vi "Facade.vi"(0 "Data In":T4, 2 "Display State In":T2, 3 "Container State":T3) -> (6 "Data Out":T4, 7 "Display State Out":T2, 8 "Action":T1)   [LabVIEW 2020, in "Recipe Entry.xctl"]
uses:
  Recipe Entry.xctl
  Data.ctl
  <vilib>/_xctls/Container State.ctl
  State.ctl
  <vilib>/_xctls/Action.ctl
  <vilib>/_xctls/XControlSupport.lvlib
panel:
  in  "Remove":bool
  in  "Target (°F)":dbl format="%#.3f"
  in  "Duration (HH:MM)":dbl format="%<%H:%M>t"
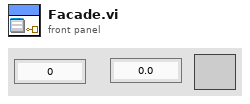
[diagram p1: front panel]
types:
  T1 = typedef "XControlSupport.lvlib/Action.ctl" = cluster{"Data Changed?":bool, "State Changed?":bool, "Action Name":string}
  T2 = typedef "Recipe Entry.xctl/State.ctl" = cluster{"Numeric":dbl}
  T3 = typedef "XControlSupport.lvlib/Container State.ctl" = cluster{"Indicator?":bool, "Run Mode?":bool, " Refnum":refnum<vi>}
  T4 = typedef "Recipe Entry.xctl/Data.ctl" = cluster{"Target":dbl, "Duration":dbl, "Remove":bool}
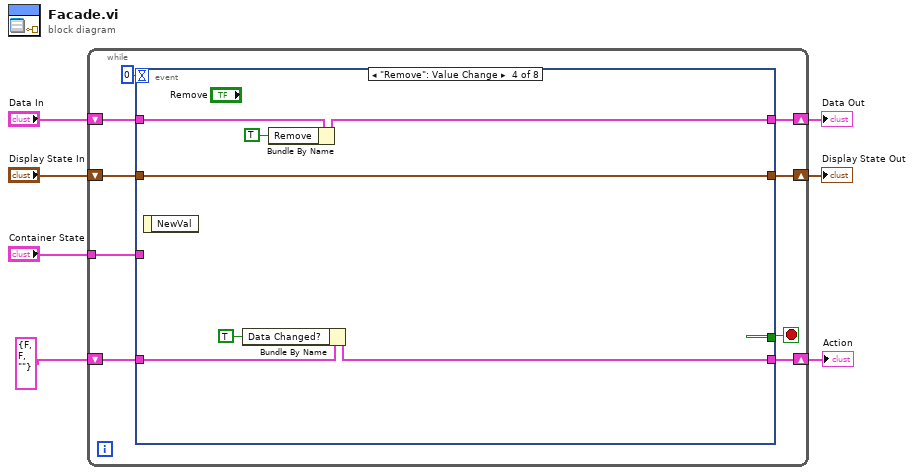
[diagram p0: block diagram]
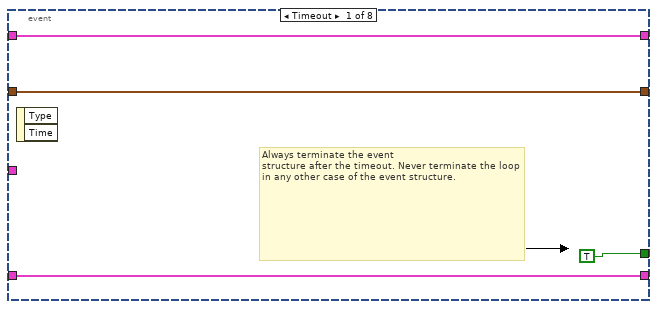
[diagram p2: hidden frame]
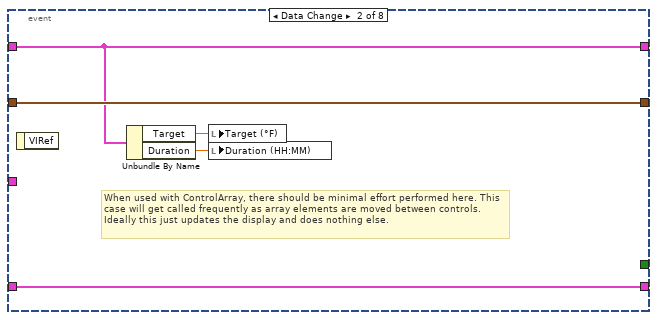
[diagram p3: hidden frame]
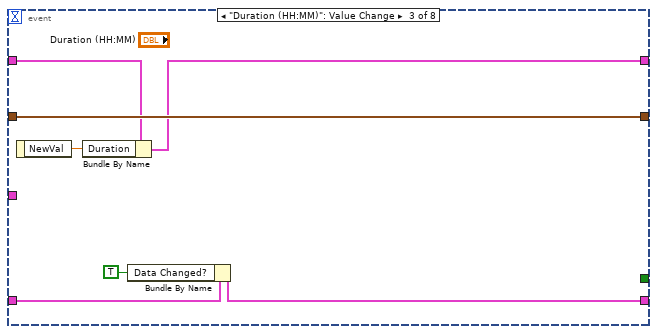
[diagram p4: hidden frame]
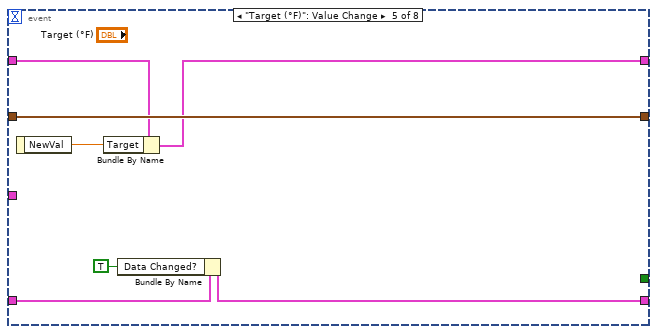
[diagram p5: hidden frame]
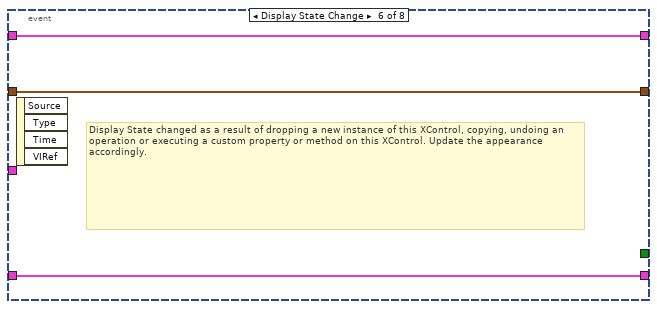
[diagram p6: hidden frame]
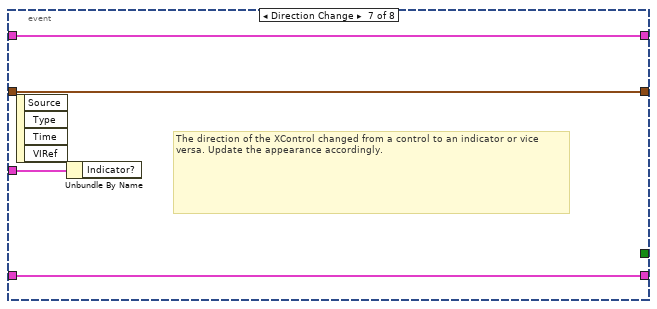
[diagram p7: hidden frame]
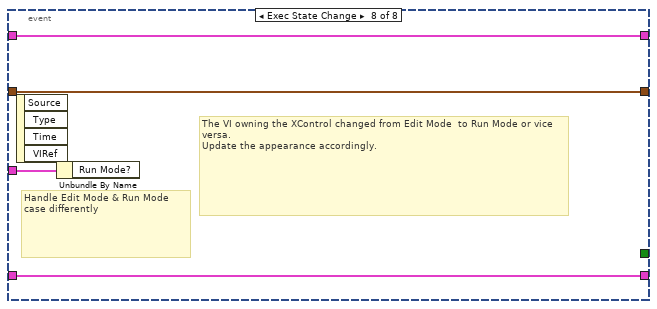
[diagram p8: hidden frame]
diagram:
  n1 = while {
    shift-right: [w15] -> w4
    shift-left: "Display State In" -> [w16]
    tunnel: "Container State" -> [w12]
    shift-right: [w10] -> w7
    shift-left: "Data In" -> [w11]
    shift-right: [w8] -> w2
    shift-left: T1 {"Data Changed?"=FALSE, "State Changed?"=FALSE, "Action Name"=""} ("Action") -> [w9]
    stop <- w14 stop-if-true
    n2 = event shown="[3] \"Remove\": Value Change" {
      selector: _ -> [_ _ _ _ _ _ _ _]
      dyn-events: _ -> [_ _ _ _ _ _ _ _]
      timeout: 0 -> [_ _ _ _ _ _ _ _]
      tunnel: w16 -> [w18 w25 w32 w39 w46 w49 w52 w56]
      tunnel: [w18 w25 w32 w39 w46 w49 w52 w56] -> w15
      tunnel: [TRUE _ _ _ _ _ _ _] -> w14
      tunnel: w12 -> [_ _ _ _ _ _ w53 w57]
      tunnel: w11 -> [w17 w23 w28 w38 w42 w48 w51 w55]
      tunnel: [w17 w23 w29 w36 w43 w48 w51 w55] -> w10
      tunnel: [w19 w24 w27 w34 w41 w47 w50 w54] -> w8
      tunnel: w9 -> [w19 w24 w31 w37 w45 w47 w50 w54]
      event Timeout {
        # "Always terminate the event\nstructure after the timeout. Never terminate the loop in any other case of the event structure."
        n3 = event-data() -> ()  [unwired: 1 in, 2 out]
      }
      event Data Change {
        # "When used with ControlArray, there should be minimal effort performed here. This case will get called frequently as array elements are moved between controls. Ideally this just updates the display and does nothing else."
        n4 = event-data() -> ()  [unwired: 1 in, 1 out]
        n5 = Unbundle By Name(w23) -> ("Target"=w22:dbl, "Duration"=w21:dbl)
        n6 = local write "Target (°F)"(w22) -> ()
        n7 = local write "Duration (HH:MM)"(w21) -> ()
      }
      event "Duration (HH:MM)": Value Change {
        n8 = event-data() -> ("NewVal"=w30:dbl)  [unwired: 1 in]
        n9 = Bundle By Name(cluster=w28, "Duration"=w30) -> (w29:T4)
        n10 = Bundle By Name(cluster=w31, "Data Changed?"=TRUE) -> (w27:T1)
      }
      event "Remove": Value Change {
        n11 = event-data() -> ()  [unwired: 1 in, 1 out]
        n12 = Bundle By Name(cluster=w37, "Data Changed?"=TRUE) -> (w34:T1)
        n13 = Bundle By Name(cluster=w38, "Remove"=TRUE) -> (w36:T4)
      }
      event "Target (°F)": Value Change {
        n14 = event-data() -> ("NewVal"=w44:dbl)  [unwired: 1 in]
        n15 = Bundle By Name(cluster=w42, "Target"=w44) -> (w43:T4)
        n16 = Bundle By Name(cluster=w45, "Data Changed?"=TRUE) -> (w41:T1)
      }
      event Display State Change {
        # "Display State changed as a result of dropping a new instance of this XControl, copying, undoing an operation or executing a custom property or method on this XControl. Update the appearance accordingly."
        n17 = event-data() -> ()  [unwired: 1 in, 4 out]
      }
      event Direction Change {
        # "The direction of the XControl changed from a control to an indicator or vice versa. Update the appearance accordingly."
        n18 = event-data() -> ()  [unwired: 1 in, 4 out]
        n19 = Unbundle By Name(w53) -> ()  [unwired: 1 out]
      }
      event Exec State Change {
        # "The VI owning the XControl changed from Edit Mode  to Run Mode or vice versa.\nUpdate the appearance accordingly."
        # "Handle Edit Mode & Run Mode\ncase differently"
        n20 = event-data() -> ()  [unwired: 1 in, 4 out]
        n21 = Unbundle By Name(w57) -> ()  [unwired: 1 out]
      }
    }
  }
  "Display State Out" <- w4
  "Data Out" <- w7
  "Action" <- w2
